vi "while.vi"() -> ()   [LabVIEW 2020]
panel:
  out "Numeric 2":u16
  in  "Knob":u16(knob) scale=0.0..100.0
  out "Thermometer":u16(slide) scale=0.0..100.0
  out "Numeric":i32
  in  "stop":bool
  # "While"
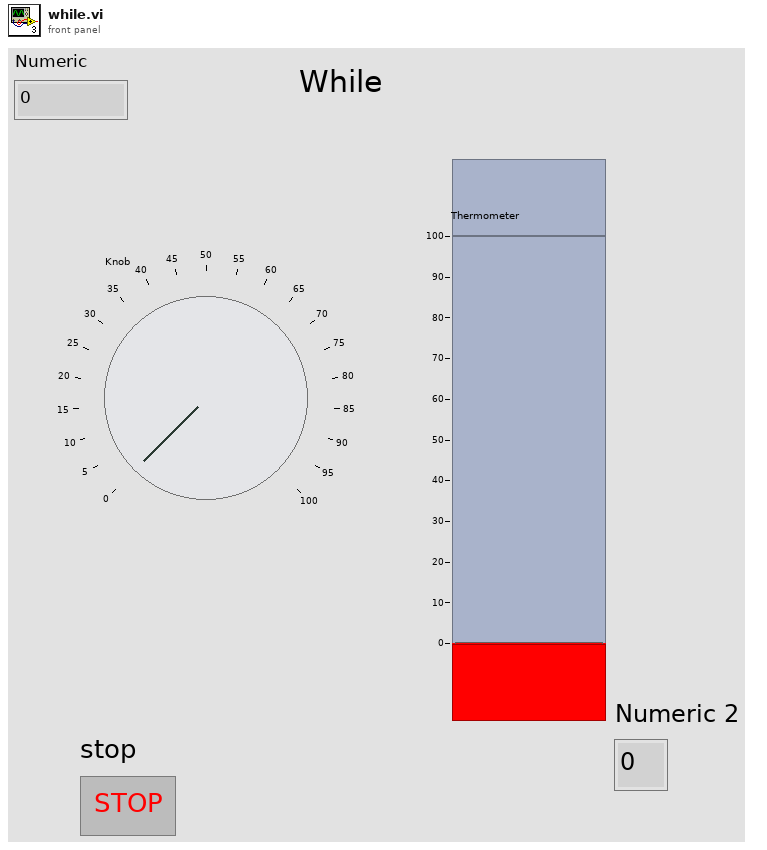
[diagram p1: front panel]
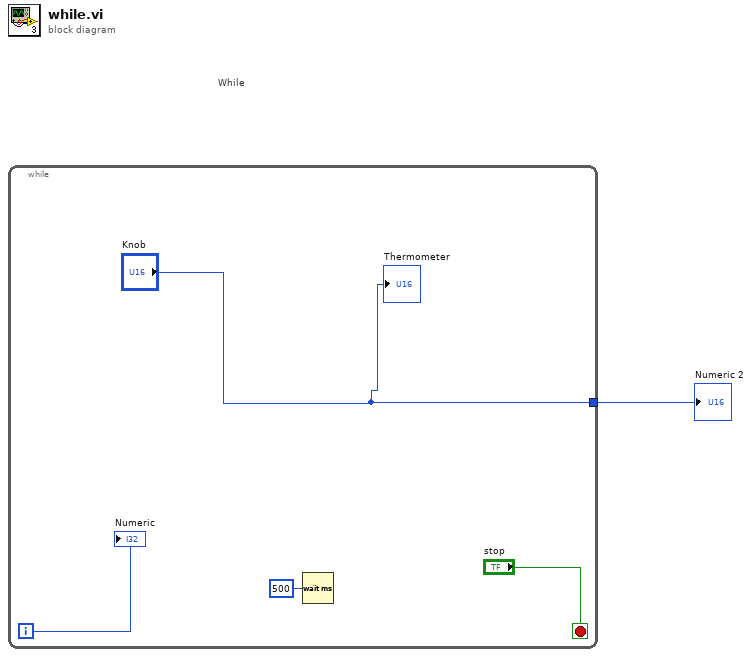
[diagram p0: block diagram]
diagram:
  # "While"
  n1 = while {
    tunnel: ["Knob"] -> w1
    i -> [w4]
    stop <- "stop" stop-if-true
    n2 = Wait (ms)(milliseconds to wait=u32 500) -> ()  [unwired: 1 out]
    "Numeric" <- w4
    "Thermometer" <- "Knob"
  }
  "Numeric 2" <- w1
